vi "GlobalLoadedParams.vi"() -> ()   [LabVIEW 2015]
panel:
  in  "display speed":string[](array[combo])
  out "display canID":dbl[](array[numeric])
  out "viewingaddress":dbl[](array[numeric])
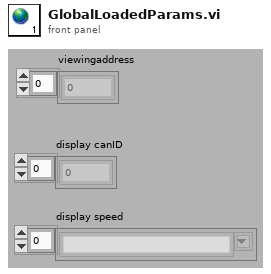
[diagram p1: front panel]
diagram:
